vi "Revision Query.vi"(7 "Address":u16, 8 "Error In":errorcluster, 11 "VISA Resource in":refnum<visa-resource-name>) -> (0 "Error Out":errorcluster, 1 "Instrument Firmware Revision":string, 2 "Instrument Driver Revision":string, 3 "VISA Resource out":refnum<visa-resource-name>)   [LabVIEW 2014, in "KIT QV.lvlib"]
doc: "Queries the current instrument firmware revision and instrument driver revision.\n\nRefer to the Readme file for detailed driver information including modification history."
uses:
  <instrlib>/KIT QV/KIT QV.lvlib
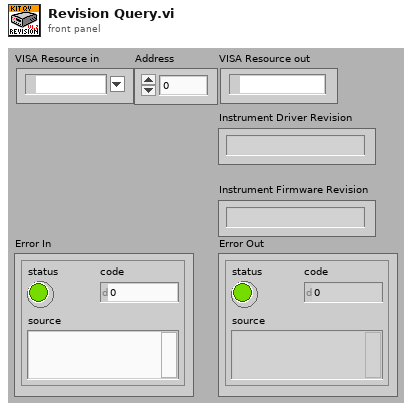
[diagram p1: front panel]
types:
  T1 = cluster{"Major":u16, "Minor":u16, "Fix":u16, "Build":u16}
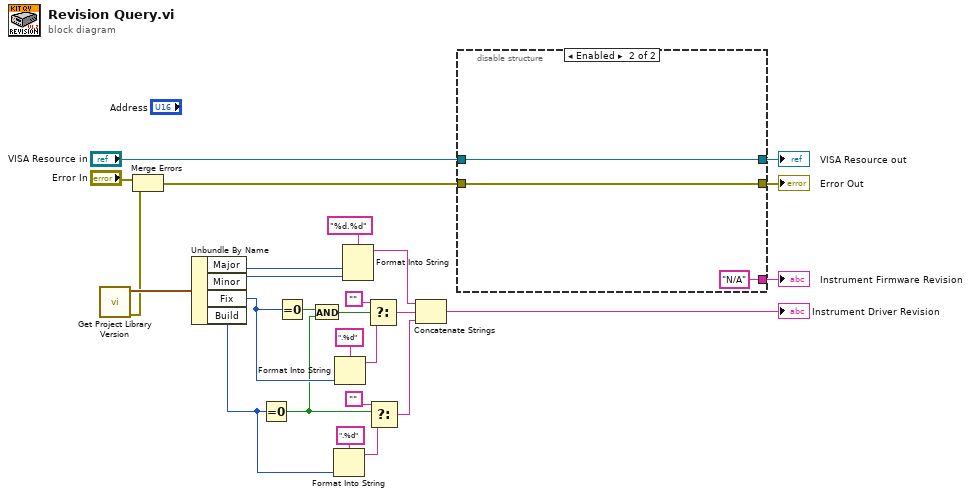
[diagram p0: block diagram]
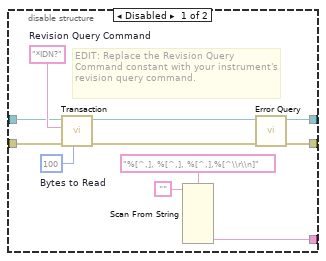
[diagram p2: hidden frame]
diagram:
  n1 = call <vilib>:"Get Project Library Version.vi"() -> ("error out"=w2:errorcluster, "Project Library Version"=w4:T1)  [unwired: 10 in]
  n2 = Merge Errors("Error In", w2) -> (w1:errorcluster)
  n3 = Unbundle By Name(w4) -> ("Major"=w11:u16, "Minor"=w10:u16, "Fix"=w8:u16, "Build"=w9:u16)
  n4 = Equal To 0?(x=w9) -> (x = 0?=w6:bool)
  n5 = Equal To 0?(x=w8) -> (x = 0?=w7:bool)
  n6 = And(x=w7, y=w6) -> (x .and. y?=w5:bool)
  n7 = Format Into String(format string=".%d", w9) -> (resulting string=w15:string)  [unwired: 2 in, 1 out]
  n8 = Format Into String(format string=".%d", w8) -> (resulting string=w19:string)  [unwired: 2 in, 1 out]
  n9 = Format Into String(format string="%d.%d", w11, w10) -> (resulting string=w17:string)  [unwired: 2 in, 1 out]
  n10 = Select(t="", s=w5, f=w19) -> (s? t:f=w16:string)
  n11 = Select(t="", s=w6, f=w15) -> (s? t:f=w12:string)
  n12 = Concatenate Strings(w17, w16, w12) -> (→"Instrument Driver Revision":string)
  n13 = disable-structure shown="Enabled" {
    disable-tunnel: [w37 "N/A" ("Instrument Firmware Revision")] -> w26
    disable-tunnel: [w35 w39] -> w25
    disable-tunnel: [w34 w38] -> w24
    disable-tunnel: "VISA Resource in" -> [w30 w39]
    disable-tunnel: w1 -> [w29 w38]
    frame Disabled {
      w33 = "*IDN?"  # Revision Query Command
      w28 = u32 100  # Bytes to Read
      # "EDIT: Replace the Revision Query Command constant with your instrument's revision query command."
      n14 = call <instrlib>:"Transaction.vi"("Bytes to Read (100)"=w28, "error in (no error)"=w29, "Command"=w33, "VISA Resource in"=w30) -> ("error out"=w32:errorcluster, "VISA Resource out"=w31:refnum<visa-resource-name>)  [unwired: 5 in, 1 out]
      n15 = Scan From String(format string="%[^,], %[^,], %[^,],%[^\\r\\n]", input string="") -> (output 4=w37:string)  [unwired: 9 in, 3 out]
      n16 = call <instrlib>:"Error Query.vi"("Error in"=w32, "VISA Resource in"=w31) -> ("Error Out"=w34:errorcluster, "VISA Resource in"=w35:refnum<visa-resource-name>)  [unwired: 6 in, 2 out]
    }
    frame Enabled {
    }
  }
  "Instrument Firmware Revision" <- w26
  "VISA Resource out" <- w25
  "Error Out" <- w24
